vi "AllDigitalStand_Digital.vi"(8 "error in (no error)":errorcluster, 10 "PFI 0 digital clock frequency":dbl=500000.0) -> (0 "error out":errorcluster, 2 "AllDigitalStand":digitalwaveform[](array[waveform]))   [LabVIEW 2018]
uses:
  <vilib>/Waveform/DWDTOps.llb/DWDT Boolean Array to Digital.vi
panel:
  in  "Window size for layer index":dbl=0.5
  in  "Steps per volume":dbl=25.0
  in  "AO Sampling rate":dbl=500000.0
  in  "stand Z vol Backward samp info":cluster{"Fs":dbl, "#s":dbl}={"Fs"=1000000.0, "#s"=136842.0}
  in  "stand Z vol Acquisition samp info":cluster{"Fs":dbl, "#s":dbl}={"Fs"=1000000.0, "#s"=263158.0}
  out "Plane indexing length":i32
  in  "Shock5 duration (s)":dbl=0.1
  in  "Shock4 duration (s)":dbl=0.01
  in  "Shock3 duration (s)":dbl=0.01
  out "Electric shock US5":bool[](array[boolean])
  out "Electric shock US4":bool[](array[boolean])
  out "Electric shock US3":bool[](array[boolean])
  in  "Shock2 duration (s)":dbl=0.001
  in  "Shock1 duration (s)":dbl=0.001
  in  "JAI camera fps":dbl=240.0
  in  "Time per volume (s)":dbl=0.4
  out "Violet evoked digital output":bool[](array[boolean])
  out "Electric shock US2":bool[](array[boolean])
  out "Electric shock US":bool[](array[boolean])
  out "PreVIEW":digitalwaveform[](graph)
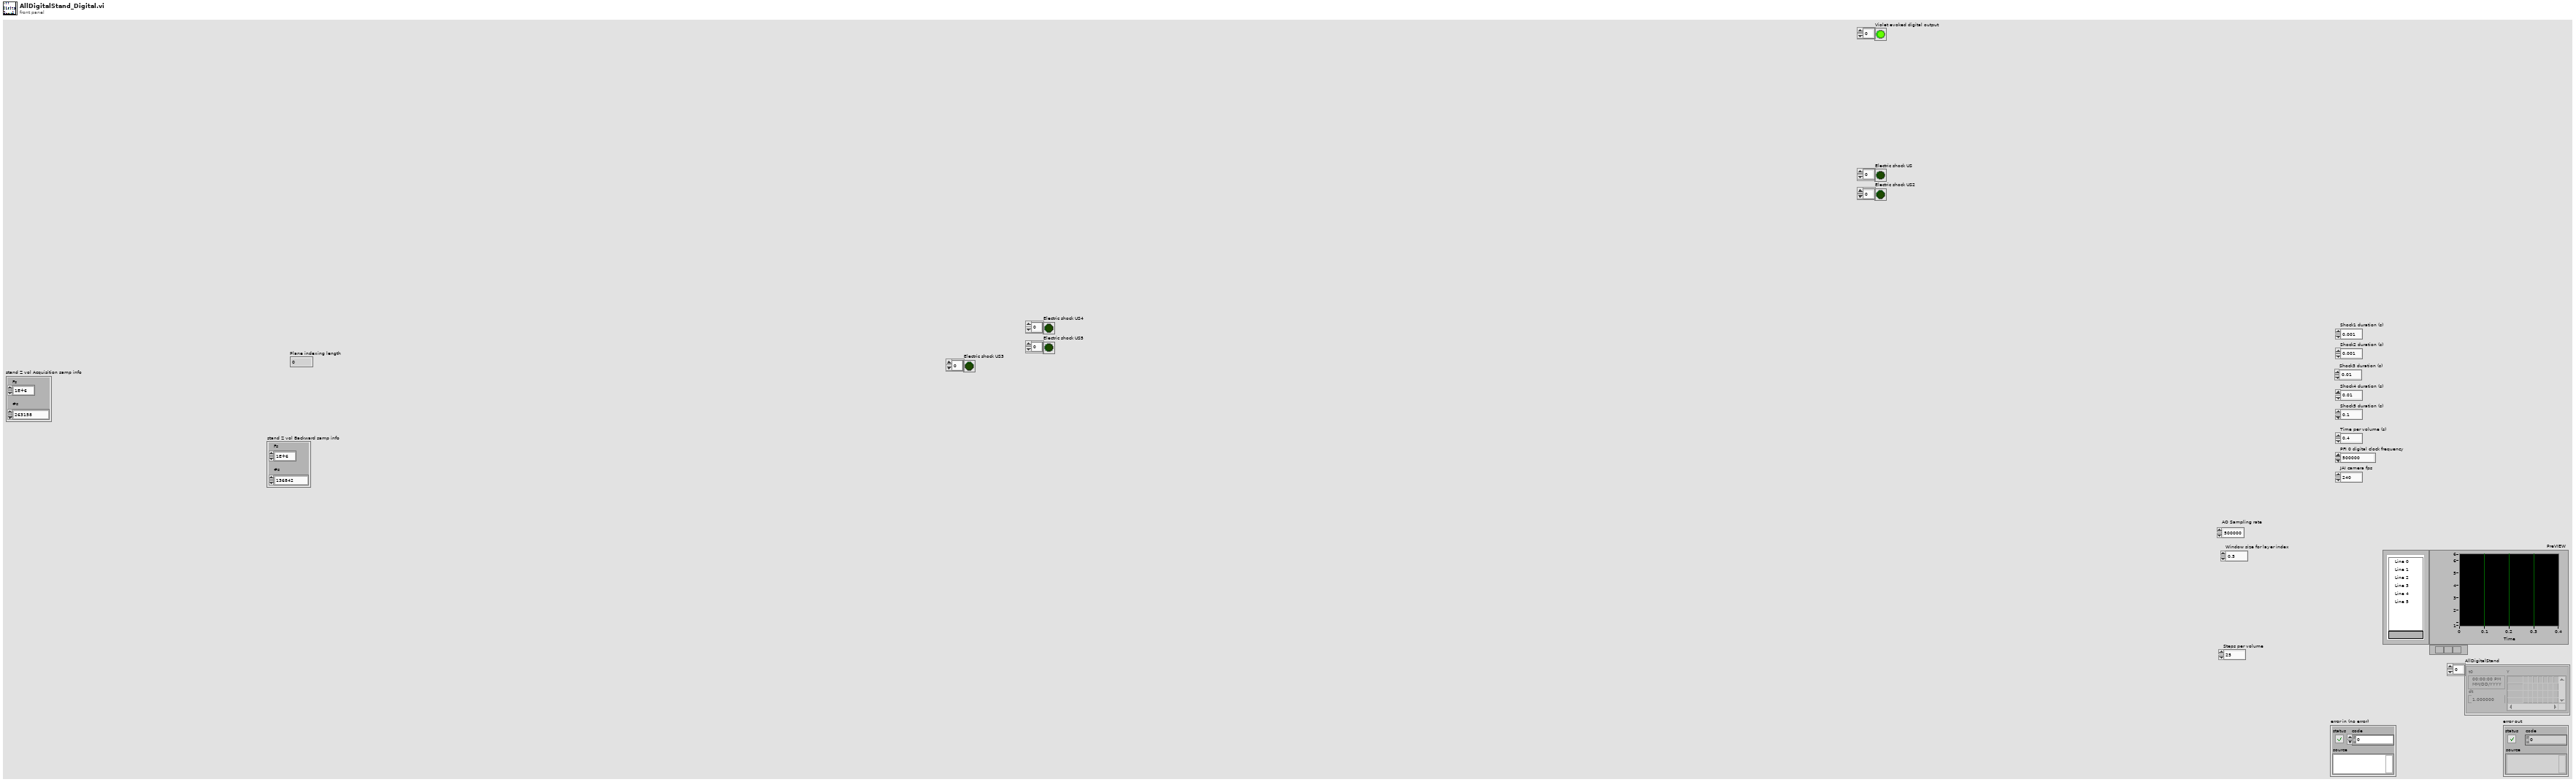
[diagram p1: front panel]
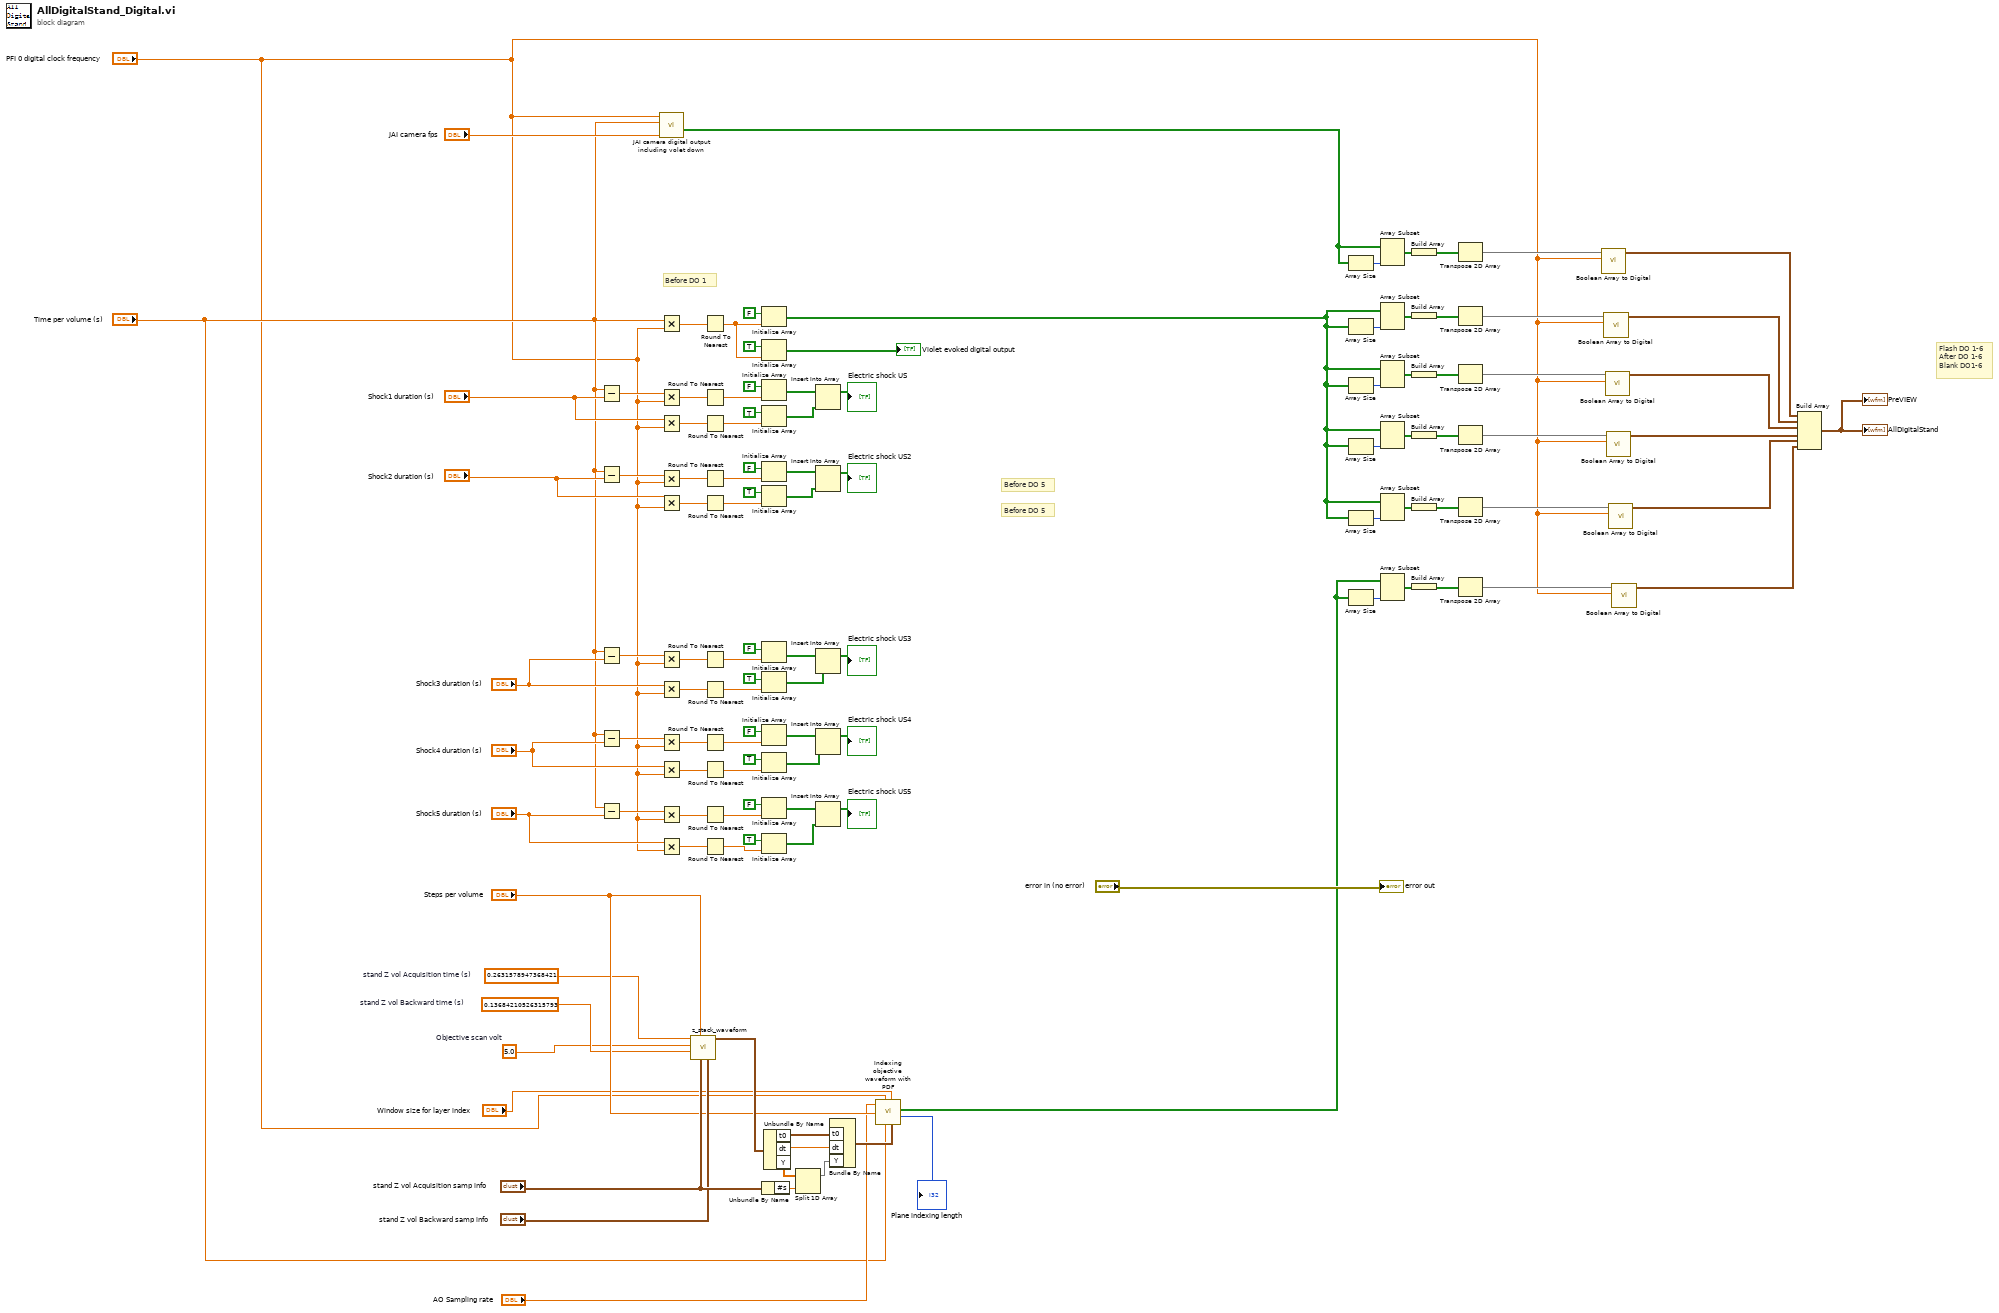
[diagram p0: block diagram]
diagram:
  w2 = 5.0  # Objective scan volt
  w4 = 0.13684210526315793  # stand Z vol Backward time (s)
  w5 = 0.2631578947368421  # stand Z vol Acquisition time (s)
  # "Before DO 5"
  # "Before DO 5"
  # "Before DO 1"
  # "Flash DO 1-6\nAfter DO 1-6\nBlank DO1-6"
  n1 = Subtract(x="Time per volume (s)", y="Shock1 duration (s)") -> (x-y=w77:dbl)
  n2 = Subtract(x="Time per volume (s)", y="Shock2 duration (s)") -> (x-y=w76:dbl)
  n3 = Subtract(x="Time per volume (s)", y="Shock3 duration (s)") -> (x-y=w46:dbl)
  n4 = Subtract(x="Time per volume (s)", y="Shock4 duration (s)") -> (x-y=w45:dbl)
  n5 = Subtract(x="Time per volume (s)", y="Shock5 duration (s)") -> (x-y=w44:dbl)
  n6 = call "JAI camera digital output including volet down.vi"("JAI camera fps"="JAI camera fps", "OG volAcquisitionTime"="Time per volume (s)", "PFI 0 digital clock frequency"="PFI 0 digital clock frequency") -> ("JAI camera digital output"=w57:bool[])  [unwired: 8 in]
  n7 = Multiply(x="Time per volume (s)", y="PFI 0 digital clock frequency") -> (x*y=w82:dbl)
  n8 = Multiply(x=w77, y="PFI 0 digital clock frequency") -> (x*y=w81:dbl)
  n9 = Multiply(x="Shock1 duration (s)", y="PFI 0 digital clock frequency") -> (x*y=w80:dbl)
  n10 = Multiply(x=w76, y="PFI 0 digital clock frequency") -> (x*y=w79:dbl)
  n11 = Multiply(x="Shock2 duration (s)", y="PFI 0 digital clock frequency") -> (x*y=w78:dbl)
  n12 = Multiply(x=w46, y="PFI 0 digital clock frequency") -> (x*y=w52:dbl)
  n13 = Multiply(x="Shock3 duration (s)", y="PFI 0 digital clock frequency") -> (x*y=w51:dbl)
  n14 = Multiply(x=w45, y="PFI 0 digital clock frequency") -> (x*y=w50:dbl)
  n15 = Multiply(x="Shock4 duration (s)", y="PFI 0 digital clock frequency") -> (x*y=w49:dbl)
  n16 = Multiply(x=w44, y="PFI 0 digital clock frequency") -> (x*y=w48:dbl)
  n17 = Multiply(x="Shock5 duration (s)", y="PFI 0 digital clock frequency") -> (x*y=w47:dbl)
  n18 = call "z_stack_waveform.vi"("Z stack backward"="stand Z vol Backward samp info", "Z stack acquisition"="stand Z vol Acquisition samp info", "Steps per Volume"="Steps per volume", "Backward Time (s)"=w4, "SPECIFIC scan volt"=w2, "Aquisition Time (s)"=w5) -> ("WaveformOut"=w19:waveform(dbl))  [unwired: 5 in]
  n19 = Round To Nearest(number=w82) -> (nearest integer value=w73:dbl)
  n20 = Round To Nearest(number=w81) -> (nearest integer value=w75:dbl)
  n21 = Round To Nearest(number=w80) -> (nearest integer value=w74:dbl)
  n22 = Round To Nearest(number=w79) -> (nearest integer value=w72:dbl)
  n23 = Round To Nearest(number=w78) -> (nearest integer value=w71:dbl)
  n24 = Round To Nearest(number=w52) -> (nearest integer value=w43:dbl)
  n25 = Round To Nearest(number=w51) -> (nearest integer value=w42:dbl)
  n26 = Round To Nearest(number=w50) -> (nearest integer value=w41:dbl)
  n27 = Round To Nearest(number=w49) -> (nearest integer value=w40:dbl)
  n28 = Round To Nearest(number=w48) -> (nearest integer value=w39:dbl)
  n29 = Round To Nearest(number=w47) -> (nearest integer value=w38:dbl)
  n30 = Initialize Array(FALSE, w73) -> (w56:bool[])
  n31 = Initialize Array(TRUE, w73) -> (→"Violet evoked digital output":bool[])
  n32 = Initialize Array(FALSE, w75) -> (w63:bool[])
  n33 = Initialize Array(TRUE, w74) -> (w64:bool[])
  n34 = Initialize Array(FALSE, w72) -> (w62:bool[])
  n35 = Initialize Array(TRUE, w71) -> (w61:bool[])
  n36 = Initialize Array(FALSE, w43) -> (w27:bool[])
  n37 = Initialize Array(TRUE, w42) -> (w26:bool[])
  n38 = Initialize Array(FALSE, w41) -> (w29:bool[])
  n39 = Initialize Array(TRUE, w40) -> (w28:bool[])
  n40 = Initialize Array(FALSE, w39) -> (w31:bool[])
  n41 = Initialize Array(TRUE, w38) -> (w30:bool[])
  n42 = Unbundle By Name("stand Z vol Acquisition samp info") -> ("#s"=w15:dbl)
  n43 = Unbundle By Name(w19) -> ("t0"=w18:timestamp, "dt"=w17:dbl, "Y"=w16:dbl[])
  n44 = Split 1D Array(array=w16, index=w15) -> (first subarray=w14:dbl[])  [unwired: 1 out]
  n45 = Insert Into Array(array=w63, new element=w64) -> (→"Electric shock US":bool[])  [unwired: 1 in]
  n46 = Insert Into Array(array=w62, new element=w61) -> (→"Electric shock US2":bool[])  [unwired: 1 in]
  n47 = Insert Into Array(array=w27, new element=w26) -> (→"Electric shock US3":bool[])  [unwired: 1 in]
  n48 = Insert Into Array(array=w29, new element=w28) -> (→"Electric shock US4":bool[])  [unwired: 1 in]
  n49 = Insert Into Array(array=w31, new element=w30) -> (→"Electric shock US5":bool[])  [unwired: 1 in]
  n50 = Bundle By Name("t0"=w18, "dt"=w17, "Y"=w14) -> (w12:waveform(dbl))  [unwired: 1 in]
  n51 = call "Indexing objective waveform with PDF.vi"("AO sampling rate"="AO Sampling rate", "PFI0 digital clock frequency"="PFI 0 digital clock frequency", "Steps per Volume"="Steps per volume", "Time per volume (s)"="Time per volume (s)", "Window size for layer index (ms)"="Window size for layer index", "Steps Waveform"=w12) -> ("Plane Indexing data"=w11:bool[], "size(s)"=→"Plane indexing length":i32)  [unwired: 3 in]
  n52 = Array Size(array=w57) -> (size(s)=w96:i32)
  n53 = Array Size(array=w56) -> (size(s)=w93:i32)
  n54 = Array Size(array=w56) -> (size(s)=w90:i32)
  n55 = Array Size(array=w56) -> (size(s)=w87:i32)
  n56 = Array Size(array=w56) -> (size(s)=w84:i32)
  n57 = Array Size(array=w11) -> (size(s)=w104:i32)
  n58 = Array Subset(array=w57, length=w96) -> (w97:bool[])  [unwired: 1 in]
  n59 = Array Subset(array=w56, length=w93) -> (w94:bool[])  [unwired: 1 in]
  n60 = Array Subset(array=w56, length=w90) -> (w91:bool[])  [unwired: 1 in]
  n61 = Array Subset(array=w56, length=w87) -> (w88:bool[])  [unwired: 1 in]
  n62 = Array Subset(array=w56, length=w84) -> (w85:bool[])  [unwired: 1 in]
  n63 = Array Subset(array=w11, length=w104) -> (w103:bool[])  [unwired: 1 in]
  n64 = Build Array(w97) -> (w95:bool[][])
  n65 = Build Array(w94) -> (w92:bool[][])
  n66 = Build Array(w91) -> (w89:bool[][])
  n67 = Build Array(w88) -> (w86:bool[][])
  n68 = Build Array(w85) -> (w83:bool[][])
  n69 = Build Array(w103) -> (w102:bool[][])
  n70 = Transpose 2D Array(2D array=w95) -> (transposed array=w108:bool[][])
  n71 = Transpose 2D Array(2D array=w92) -> (transposed array=w109:bool[][])
  n72 = Transpose 2D Array(2D array=w89) -> (transposed array=w110:bool[][])
  n73 = Transpose 2D Array(2D array=w86) -> (transposed array=w111:bool[][])
  n74 = Transpose 2D Array(2D array=w83) -> (transposed array=w112:bool[][])
  n75 = Transpose 2D Array(2D array=w102) -> (transposed array=w105:bool[][])
  n76 = call-poly <vilib>:"Boolean Array to Digital.vi"("sample rate"="PFI 0 digital clock frequency", "boolean array"=w108) -> ("digital waveform"=w98:digitalwaveform)  [unwired: 8 in, 1 out]
  n77 = call-poly <vilib>:"Boolean Array to Digital.vi"("sample rate"="PFI 0 digital clock frequency", "boolean array"=w109) -> ("digital waveform"=w107:digitalwaveform)  [unwired: 8 in, 1 out]
  n78 = call-poly <vilib>:"Boolean Array to Digital.vi"("sample rate"="PFI 0 digital clock frequency", "boolean array"=w110) -> ("digital waveform"=w106:digitalwaveform)  [unwired: 8 in, 1 out]
  n79 = call-poly <vilib>:"Boolean Array to Digital.vi"("sample rate"="PFI 0 digital clock frequency", "boolean array"=w111) -> ("digital waveform"=w113:digitalwaveform)  [unwired: 8 in, 1 out]
  n80 = call-poly <vilib>:"Boolean Array to Digital.vi"("sample rate"="PFI 0 digital clock frequency", "boolean array"=w112) -> ("digital waveform"=w100:digitalwaveform)  [unwired: 8 in, 1 out]
  n81 = call-poly <vilib>:"Boolean Array to Digital.vi"("sample rate"="PFI 0 digital clock frequency", "boolean array"=w105) -> ("digital waveform"=w99:digitalwaveform)  [unwired: 8 in, 1 out]
  n82 = Build Array(w98, w107, w106, w113, w100, w99) -> (→"PreVIEW" →"AllDigitalStand":digitalwaveform[])
  "error out" <- "error in (no error)"
